vi "OCT.vi"() -> ()   [LabVIEW 2015]
doc: "I. Description:\nThis example demonstrates how to acquire a continuous amount of data (Waveform) using the DAQ device's internal clock.\n\nII. Instructions for Running:\n1. Create an analog input voltage channel.\n2. Set the rate for the sample clock. Additionally, define the sample mode to be continuous.\n3. Call the Start VI to start the acquisition.\n4. Read the waveform data in a loop until the user hits the stop button or an error occurs.\nNote: This example reads data from one or more channels and returns an array of data. Use the Index Array function to access an individual channel of data.\n5. Call the Clear Task VI to clear the Task.\n6. Use the popup dialog box to display an error if any.\n\nIV. I/O Connections Overview:\nMake sure your signal input terminal matches the Physical Channel I/O Control. For further connection information, refer to your hardware reference manual."
uses:
  Type Defs/OCT DAQ Channel Data Type.ctl
  Type Defs/OCT Hardware States.ctl
  Classes/Galvo/Scanning Cluster.ctl
  Classes/DAQ/DAQ Parameters.ctl
  Classes/DAQ/Trigger Source.ctl
  Classes/DAQ/Trigger Slope.ctl
  Classes/DAQ/Clock Control.ctl
  Classes/Galvo/Galvo.lvclass
  Classes/Nufern/Nufern Digital Timing Control.ctl
  Classes/Processing/Intensity/Intensity Processing.lvclass
  Classes/DAQ/DAQ Card Options.ctl
  Classes/Laser/Laser Options.ctl
  Classes/D to A/External Clock Selection.ctl
  Classes/Galvo/Galvo Options.ctl
  Classes/Laser/Axsun/1310/Axsun_1310_SS.lvclass
  Classes/DAQ/ATS9350/ATS9350.lvclass
  Classes/Processing/En Face States.ctl
  Classes/DAQ/DAQ Control Functional Global States.ctl
  Classes/Nufern/Nufern Functional Global States.ctl
  Classes/Processing/Filter/Filter List.ctl
  Classes/Processing/Filter/Kernel Size.ctl
  Classes/Processing/Filter/Std_Dev_Filter/Std. Deviation.lvclass
  Classes/Processing/Filter/Filter.lvclass
  Classes/Processing/Filter/Speckle_Variance_Filter/Speckle Variance Filter.lvclass
  Classes/D to A/No Clock/No Clock.lvclass
  Classes/Galvo/NI Galvo/NI Galvo.lvclass
  Classes/Nufern/Nufern Digital Control Global.vi
  Classes/DAQ/ATS660/ATS660 Class.lvclass
  Classes/DAQ/ATS9462/ATS9462 Class.lvclass
  Classes/Laser/Santec/HSL-2000/HSL-2000.lvclass
  Classes/Laser/Insite/Insight.lvclass
  Classes/D to A/Wavepond/Wavepond.lvclass
  Classes/Galvo/No Galvos/No Galvos.lvclass
  Classes/DAQ/DAQ Class.lvclass
  Classes/Laser/Laser.lvclass
panel:
  out "Enface":T1(plugin-control)
  out "Intensity Graph":sgl[][](graph)
  in  "Nufern Digital Timing Control":T2={"Fire"=FALSE, "Start A-Scan"=0, "Stop A-Scan"=0, "Reps per Fire"=1, "B-Scan Spacing"=1} {"B-Scan Spacing" min=0 max=5000; "Reps per Fire" min=1 max=5000}
  out "Saved Galvo":refnum<class "Galvo.lvclass">
  out "AFG11000 Task":refnum<k21>
  out "Alazar Task":refnum<k21>
  out "Initial DAQ Parameters":T3={"Points Per A-Scan"=1280, "A-Scans Per B-Scan"=832, "Number of B-Scans"=1, "B-Scans Per Transfer"=2, "Trigger Voltage"=140.0, "Trigger Source"=enum."External", "Trigger Slope"=enum."Rising", "Channel"=enum."Channel 1", "Clock"=enum."External Clock", "Bits per Sample"=16.0, "Range"=4.0, "Start Trim"=140, "Stop Trim"=180}
  in  "Laser Status":string
  in  "Scanning Parameters":T8={"Fast Axis Offset"=0.0, "Slow Axis Offset"=0.0, "Slow Axis Amp"=2.0, "Fast Axis Amp"=2.0, "Scan Pattern"=enum."Raster"} {"Fast Axis Amp" max=20 format="%#.2f"; "Slow Axis Amp" max=20 format="%#.2f"; "Slow Axis Offset" max=10 format="%#.2f"; "Fast Axis Offset" max=10 format="%#.2f"}
  out "Log10?":bool
  in  "OCT Hardware States":T9
  out "Background Array":u16[](array[numeric])
  in  "Save Sweep Button":bool
  in  "Data Format":T6
  in  "Save Sweep":bool
  in  "Stop Button":bool
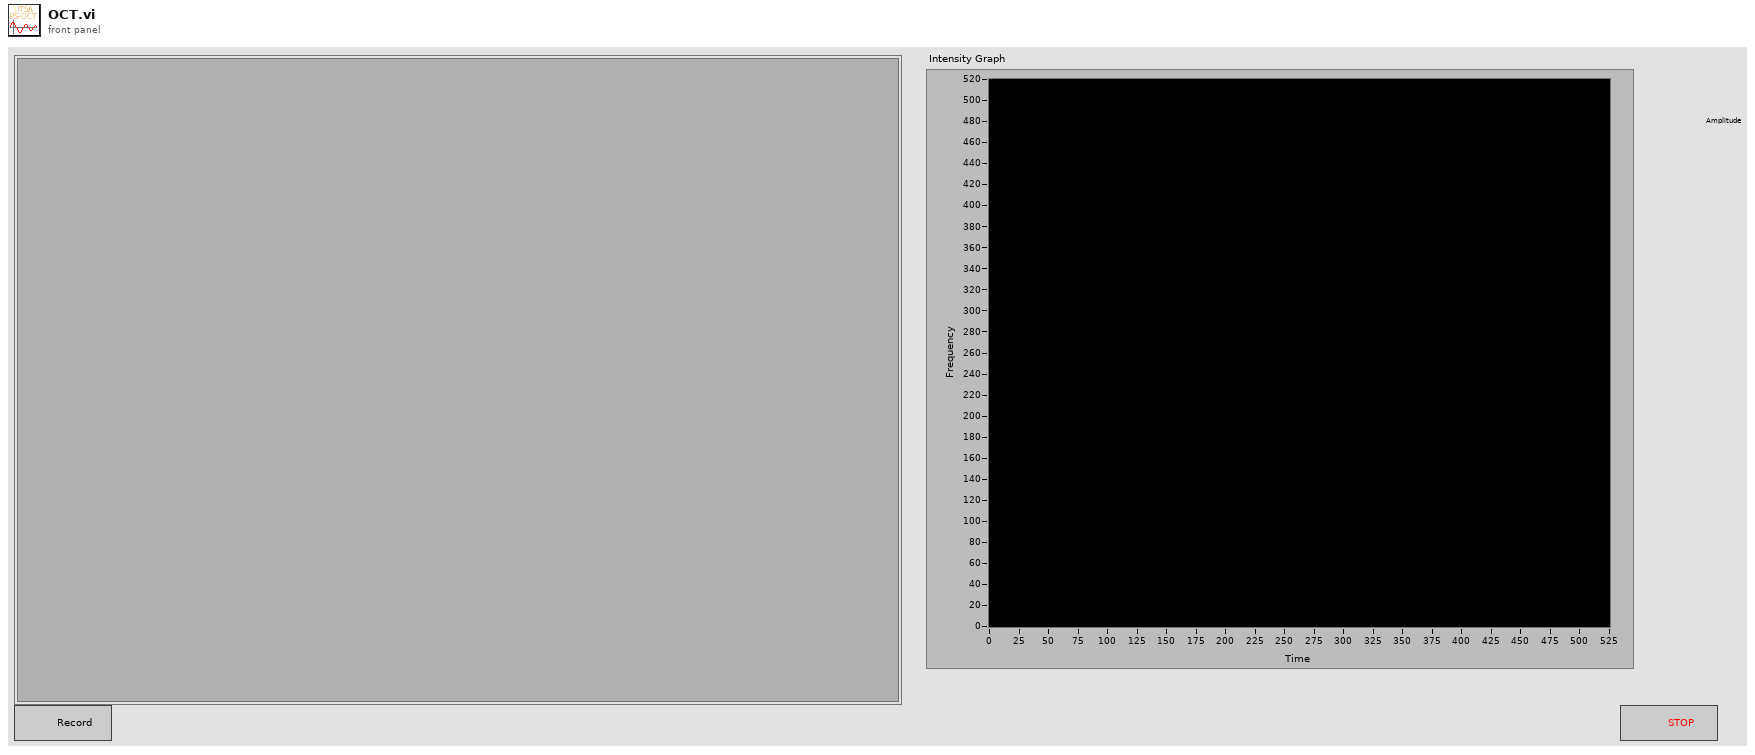
[diagram p1: front panel]
types:
  T1 = typedef "IMAQ Image.ctl" = refnum<image>
  T2 = typedef "Nufern Digital Timing Control.ctl" = cluster{"Fire":bool, "Start A-Scan":u32, "Stop A-Scan":u32, "Reps per Fire":i32, "B-Scan Spacing":i32}
  T3 = typedef "DAQ Class.lvclass/DAQ Parameters.ctl" = cluster{"Points Per A-Scan":u32, "A-Scans Per B-Scan":u32, "Number of B-Scans":u32, "B-Scans Per Transfer":u32, "Trigger Voltage":sgl, "Trigger Source":T4, "Trigger Slope":T5, "Channel":T6, "Clock":T7, "Bits per Sample":dbl, "Range":dbl, "Start Trim":u32, "Stop Trim":u32}
  T4 = typedef "DAQ Class.lvclass/Trigger Source.ctl" = enum16{"External", "Channel A", "Channel B"}
  T5 = typedef "DAQ Class.lvclass/Trigger Slope.ctl" = enum16{"Rising", "Falling"}
  T6 = typedef "OCT DAQ Channel Data Type.ctl" = enum16{"Channel 1", "Channel 2", "Channel 1 and 2"}
  T7 = typedef "DAQ Class.lvclass/Clock Control.ctl" = enum16{"Internal Clock", "External Clock"}
  T8 = typedef "Galvo.lvclass/Scanning Cluster.ctl" = cluster{"Fast Axis Offset":sgl, "Slow Axis Offset":sgl, "Slow Axis Amp":sgl, "Fast Axis Amp":sgl, "Scan Pattern":enum16{"Raster", "Triangle Raster", "Sinusoid Raster"}}
  T9 = typedef "OCT Hardware States.ctl" = enum16{"Acquire Data", "Initialize Laser", "Initialize Galvos", "Startup", "Reset DAQ", "Background Subtraction", "Acquire Background", "Update DAQ Parameters", "Stop", "Set Clock", "Initialize DAQ", "Set Resampling Array", "Save Sweep", "Configure Laser", "128 x 128", "512 x 1", "512 x 512", "Review Data", "Configure Trigger", "Update Galvos", "Update Filter", "Fire Digital Output", "Configure Digital Output", "Save Galvo Settings", "Load Galvo Settings"}
  T10 = typedef "Galvo Options.ctl" = enum16{"NI Galvos", "No Galvos"}
  T11 = typedef "External Clock Selection.ctl" = enum16{"Wavepond", "None"}
  T12 = typedef "Laser Options.ctl" = enum16{"HSL-2000", "Insight_1310", "Axsuin_1310"}
  T13 = typedef "DAQ Class.lvclass/DAQ Card Options.ctl" = enum16{"ATS660", "ATS9462", "ATS9350"}
  T14 = typedef "Nufern Functional Global States.ctl" = enum16{"Init", "Generate Waveform", "Fire", "Shutdown", "Stop"}
  T15 = typedef "DAQ Control Functional Global States.ctl" = enum16{"Status", "Set Processing Finished", "Reset", "Clear", "Set DAQ Finished"}
  T16 = typedef "Kernel Size.ctl" = enum16{"3x3", "5x5", "3x5", "5x3"}
  T17 = typedef "Filter.lvclass/Filter List.ctl" = enum16{"None", "Std. Dev.", "Speckle Variance"}
  T18 = enum32{"Invalid", "Standard", "Closed", "Hidden", "Minimized", "Maximized"}
  T19 = typedef "En Face States.ctl" = enum16{"Reset", "Update", "Get EnFace"}
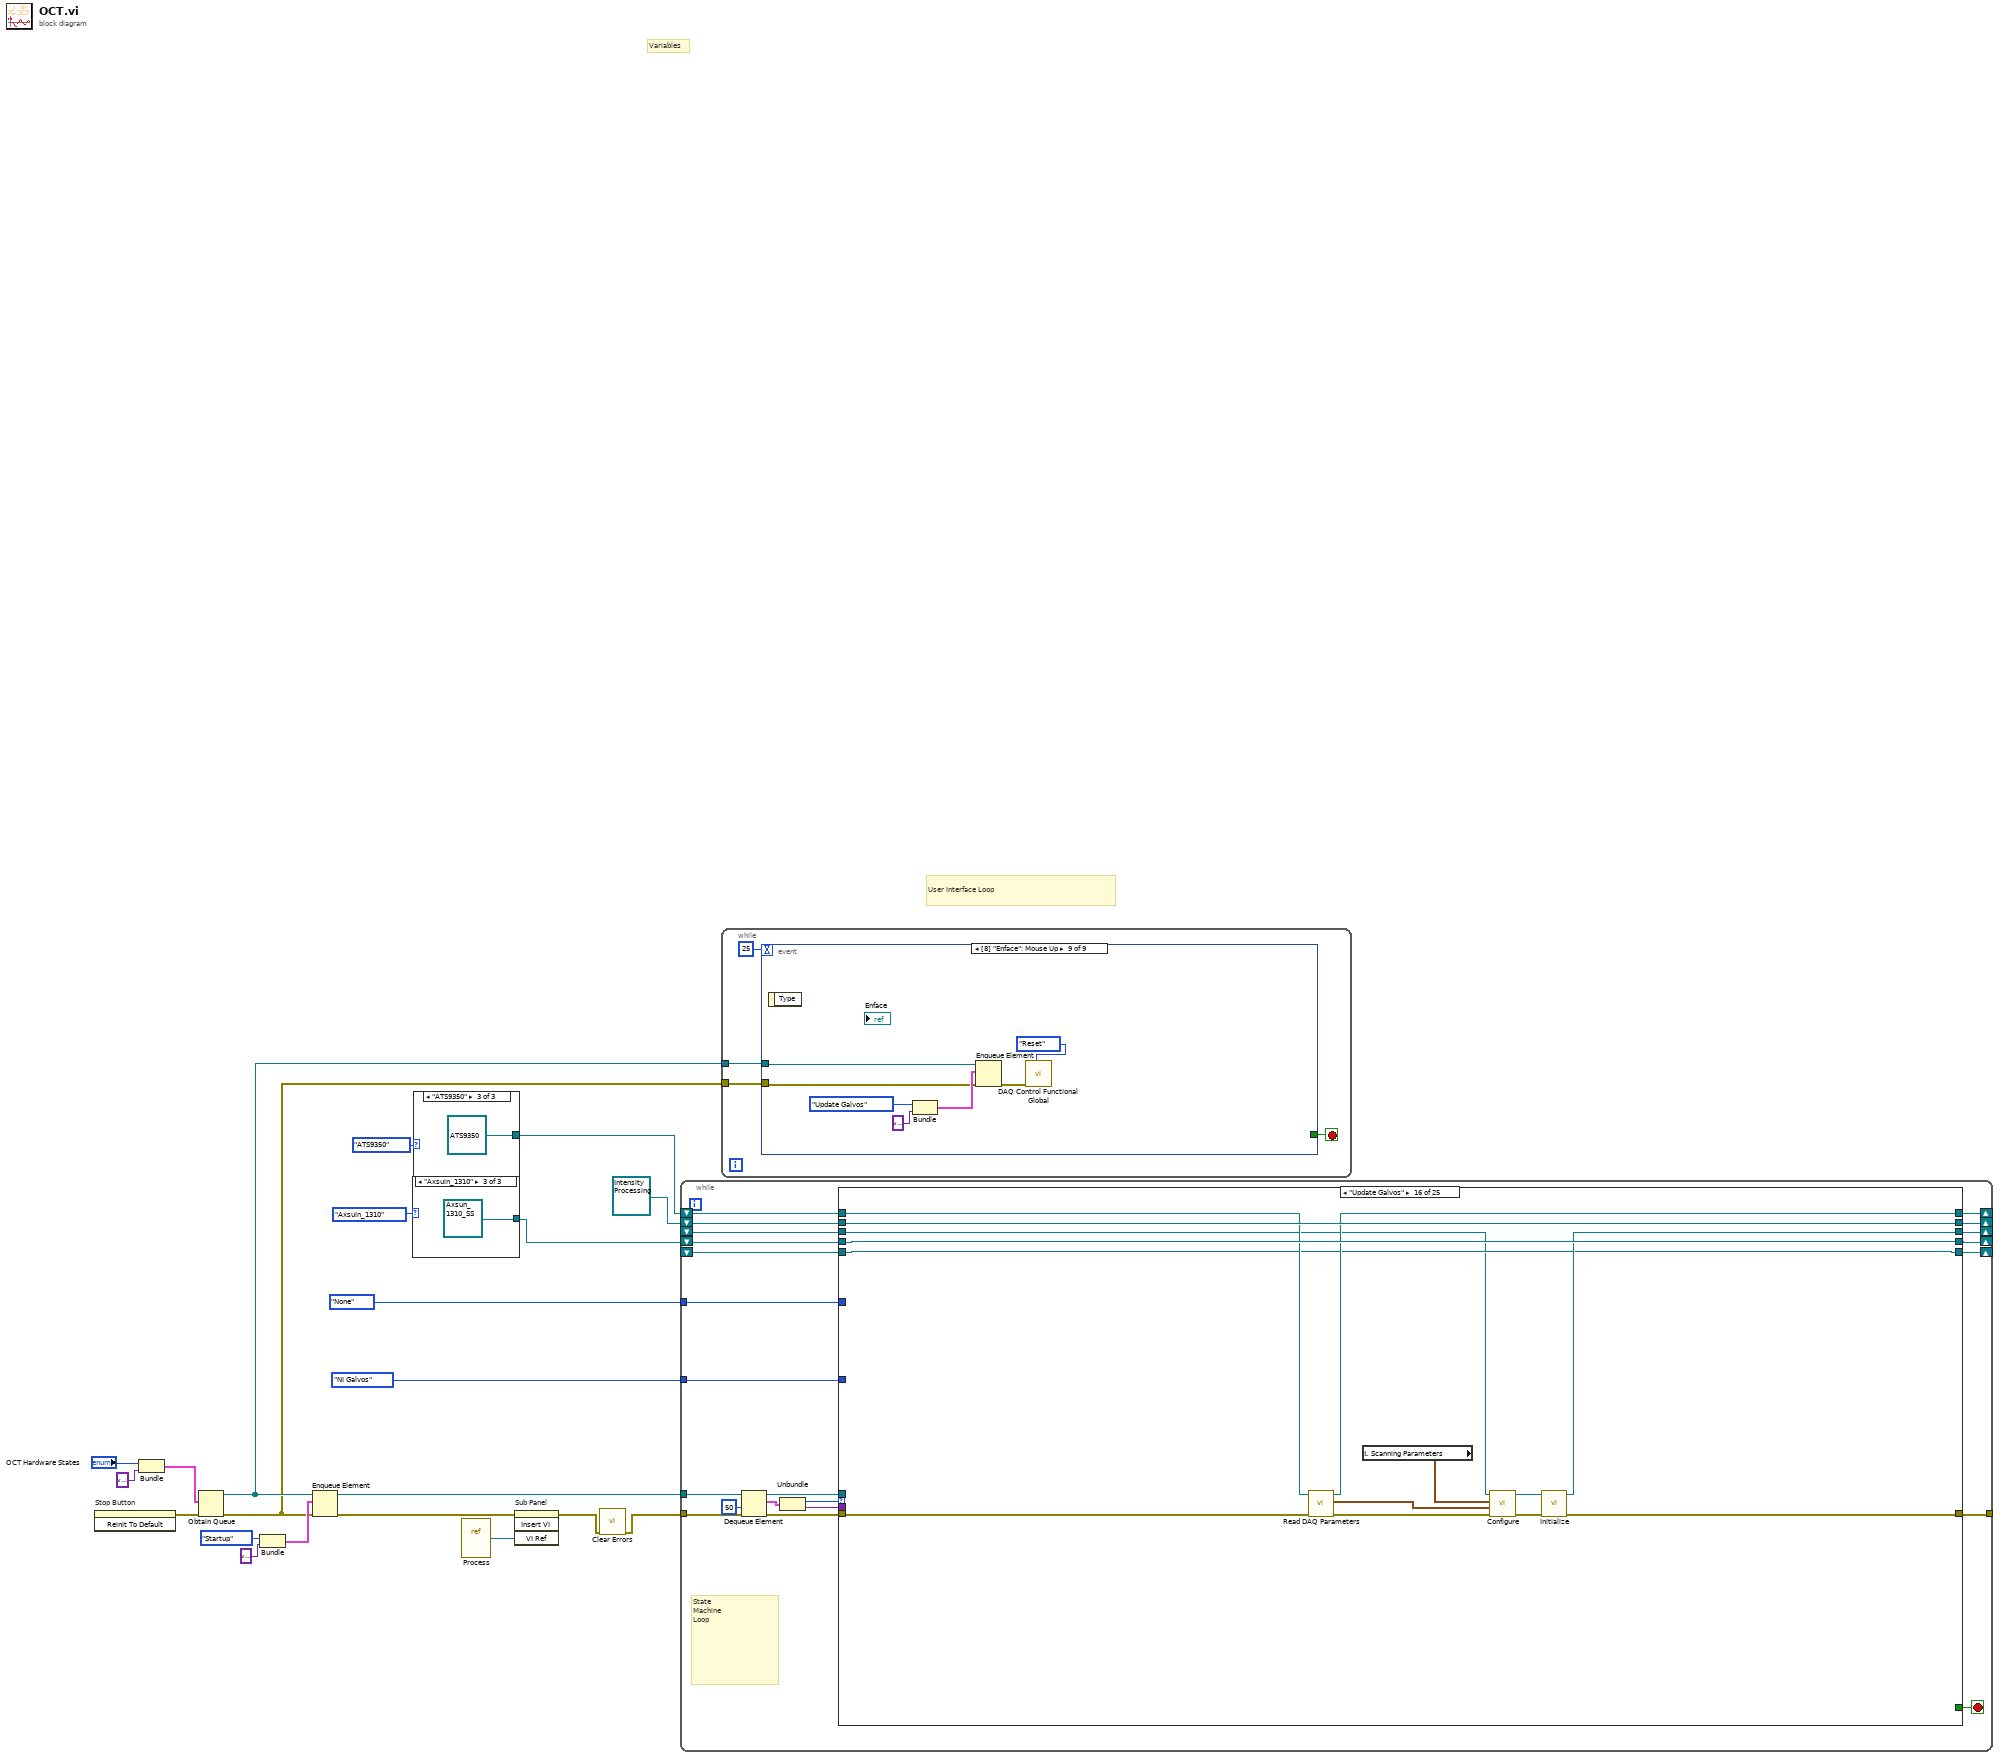
[diagram p0: block diagram]
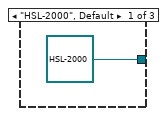
[diagram p2: hidden frame]
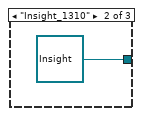
[diagram p3: hidden frame]
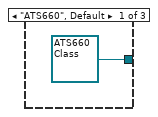
[diagram p4: hidden frame]
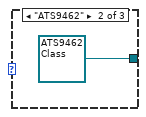
[diagram p5: hidden frame]
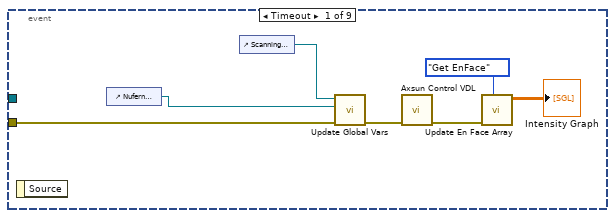
[diagram p6: hidden frame]
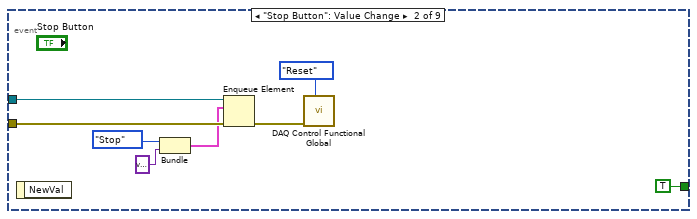
[diagram p7: hidden frame]
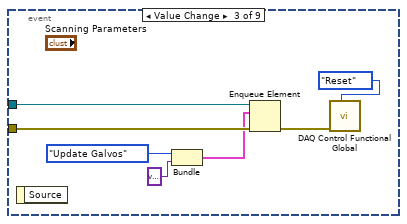
[diagram p8: hidden frame]
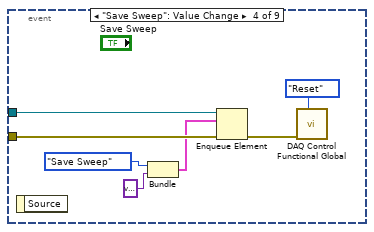
[diagram p9: hidden frame]
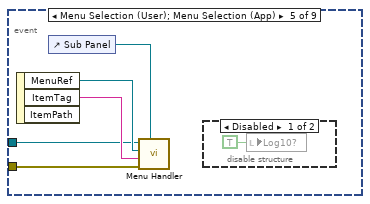
[diagram p10: hidden frame]
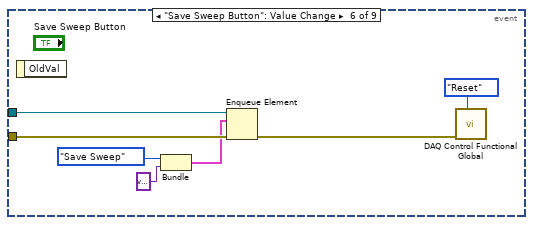
[diagram p12: hidden frame]
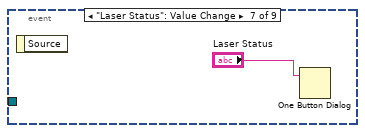
[diagram p13: hidden frame]
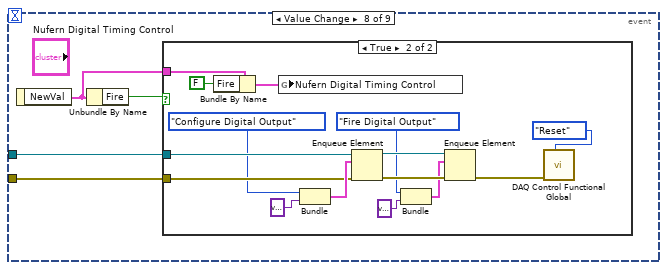
[diagram p14: hidden frame]
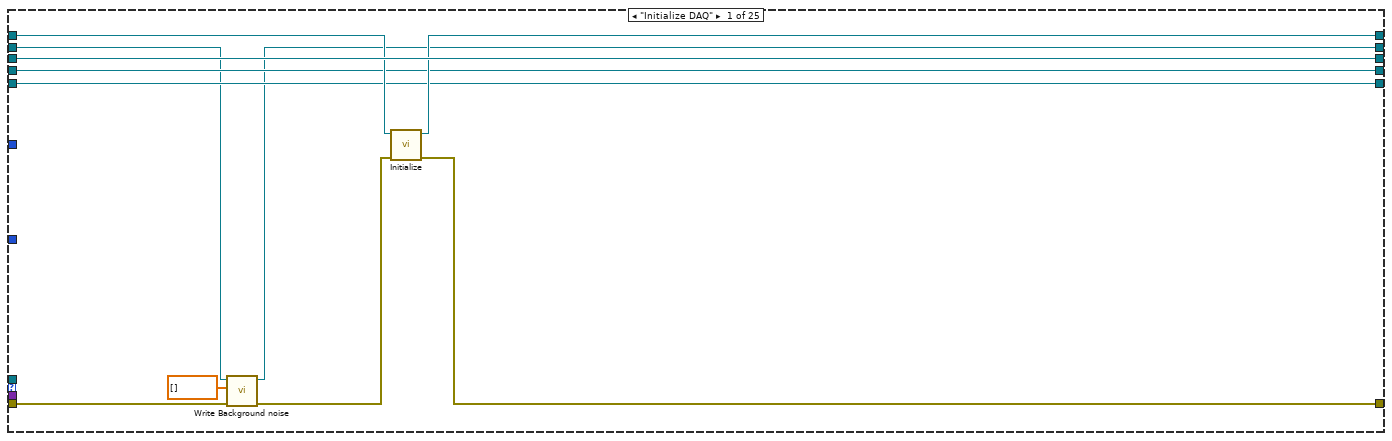
[diagram p16: hidden frame]
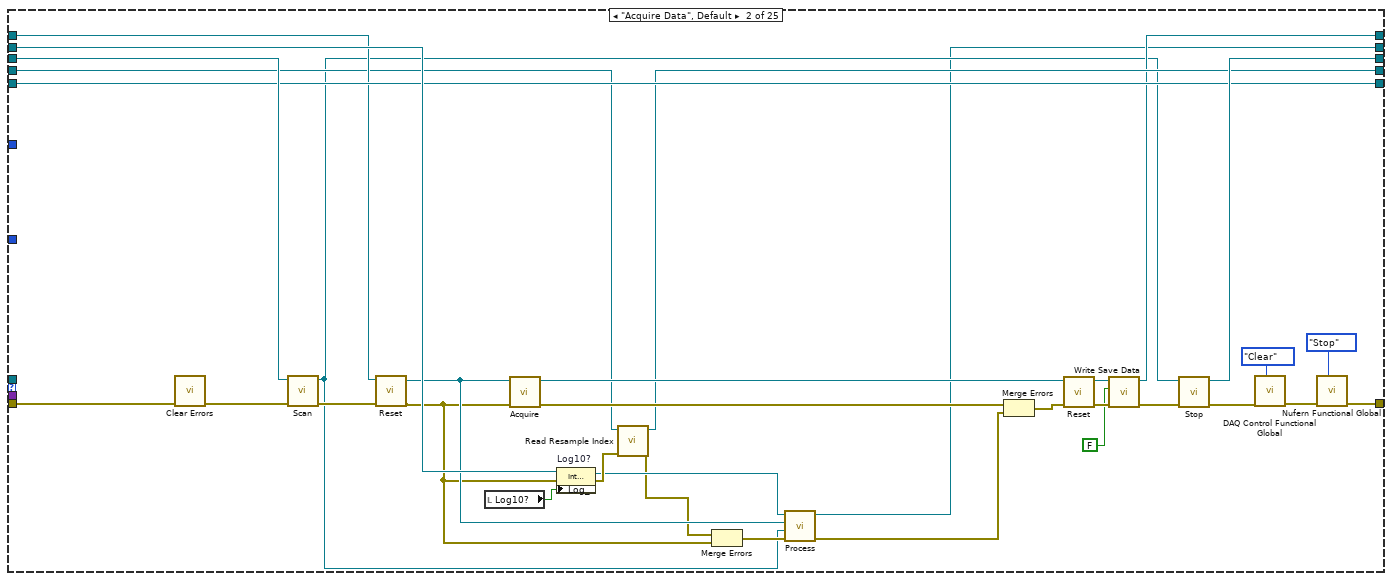
[diagram p17: hidden frame]
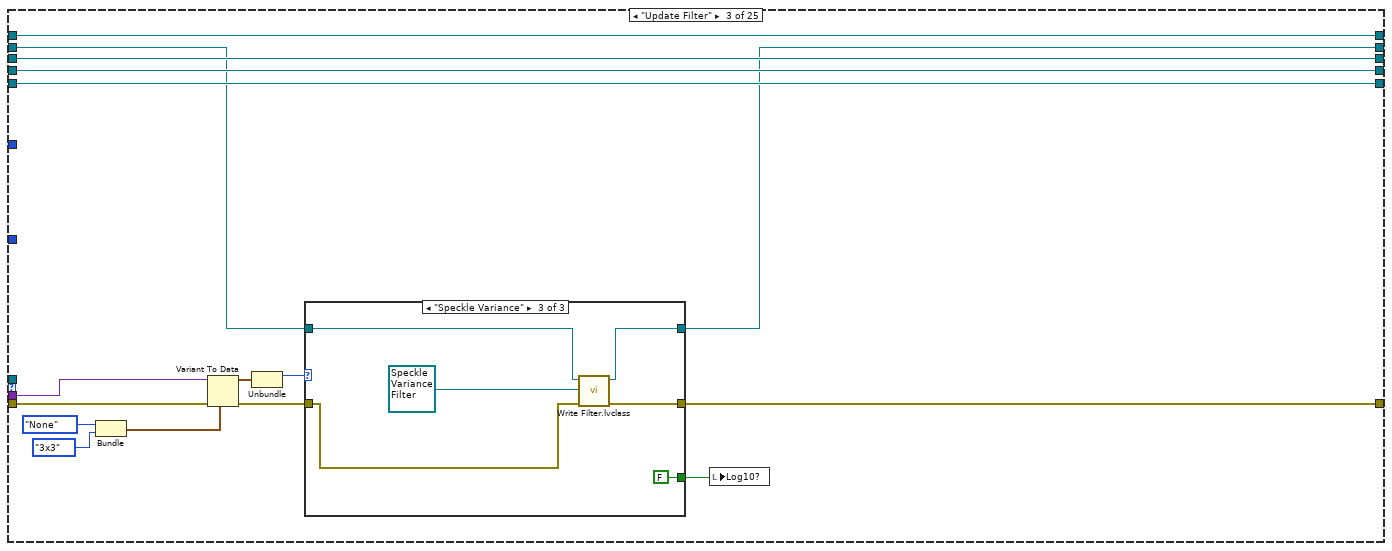
[diagram p18: hidden frame]
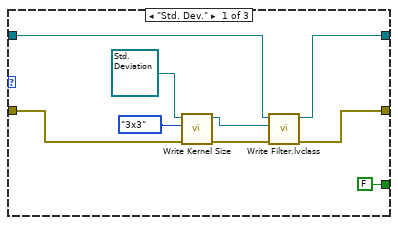
[diagram p19: hidden frame]
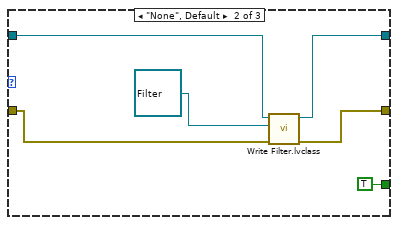
[diagram p20: hidden frame]
diagram:
  # "User Interface Loop"
  # "Variables"
  n1 = invoke on="Stop Button" class="Bool (strict)" method="Reinit To Default"() -> (error out=w14:errorcluster)  [unwired: 3 in, 2 out]
  n2 = Bundle("OCT Hardware States"="OCT Hardware States", variant) -> (w5:cluster{"OCT Hardware States":T9, variant})  [unwired: 1 in]
  n3 = Obtain Queue(element data type=w5, error in (no error)=w14) -> (queue out=w21:refnum<queue>, error out=w1:errorcluster)  [unwired: 3 in, 1 out]
  n4 = Bundle("element"=OCT_Hardware_States."Startup", variant) -> (w3:cluster{"element":T9, variant})  [unwired: 1 in]
  n5 = Enqueue Element(queue=w21, element=w3, error in (no error)=w1) -> (queue out=w18:refnum<queue>, error out=w10:errorcluster)  [unwired: 1 in, 1 out]
  n6 = case shown="\"Axsuin_1310\"" Laser_Options."Axsuin_1310" ("Laser Options") {
    tunnel: [refnum<class "HSL-2000.lvclass"> refnum ("HSL-2000.lvclass") refnum<class "Insight.lvclass"> refnum ("Insight.lvclass") refnum<class "Axsun_1310_SS.lvclass"> refnum ("Axsun_1310_SS.lvclass")] -> w15
    frame "HSL-2000", Default {
    }
    frame "Insight_1310" {
    }
    frame "Axsuin_1310" {
    }
  }
  n7 = case shown="\"ATS9350\"" DAQ_Card_Options."ATS9350" {
    tunnel: [refnum<class "ATS660 Class.lvclass"> refnum ("ATS660 Class.lvclass") refnum<class "ATS9462 Class.lvclass"> refnum ("ATS9462 Class.lvclass") refnum<class "ATS9350.lvclass"> refnum ("ATS9350.lvclass")] -> w19
    frame "ATS660", Default {
    }
    frame "ATS9462" {
    }
    frame "ATS9350" {
    }
  }
  n8 = vi-ref "Process.vi"() -> (w11:refnum<vi>)
  n9 = invoke on="Sub Panel" class="SubPanel" method="Insert VI"(error in=w10, "VI Ref"=w11) -> (error out=w9:errorcluster)  [unwired: 2 in, 3 out]
  n10 = call <vilib>:"Clear Errors.vi"("error in (no error)"=w9) -> ("error out"=w8:errorcluster)  [unwired: 5 in, 1 out]
  n11 = while {
    tunnel: w18 -> [w49]
    tunnel: w8 -> [w44]
    tunnel: [w45] -> _
    shift-right: [w42] -> _
    shift-left: w19 -> [w43]
    shift-right: [w38] -> _
    shift-left: refnum<class "Intensity Processing.lvclass"> refnum ("Intensity Processing.lvclass") -> [w41]
    shift-right: [w37] -> _
    shift-left: _ -> [w40]
    shift-right: [w36] -> _
    shift-left: w15 -> [w39]
    shift-right: [w34] -> _
    shift-left: _ -> [w33]
    tunnel: External_Clock_Selection."None" ("External Clock Options") -> [w32]
    tunnel: Galvo_Options."NI Galvos" ("Galvo Options") -> [w31]
    stop <- w35 stop-if-true
    # "State\nMachine\nLoop"
    n12 = Dequeue Element(queue=w49, timeout in ms (-1)=50, error in (no error)=w44) -> (queue out=w47:refnum<queue>, element=w30:cluster{"OCT Hardware States":T9, variant}, error out=w48:errorcluster)  [unwired: 1 out]
    n13 = Unbundle(w30) -> ("OCT Hardware States"=w29:T9, w28:variant)
    n14 = case shown="\"Update Galvos\"" w29 {
      tunnel: w48 -> [w54 w77 w105 w143 w155 w162 w179 w195 _ w241 w261 _ w336 w367 w369 w401 _ w417 w429 w437 w446 w458 w476 w488 w497]
      tunnel: w47 -> [_ _ _ w144 _ _ _ _ _ _ _ _ w337 w366 _ _ _ _ _ _ _ _ w474 _ _]
      tunnel: [w60 w64 w95 w131 w146 w167 w183 w199 _ w229 w257 _ w307 w365 w376 w408 _ w416 w424 w439 _ w457 w465 w483 w497] -> w45
      tunnel: w43 -> [w58 w81 w109 w139 w148 w163 w180 w196 w208 w232 w258 w306 w341 w364 w372 w404 w413 w421 w432 w445 w455 w463 w482 w484 w502]
      tunnel: [w57 w69 w109 w139 w147 w168 w184 w200 w208 w231 w254 w306 w341 w363 w371 w403 w413 w421 w432 w445 w455 w463 w482 w485 w502] -> w42
      tunnel: w41 -> [w51 w85 w102 w141 w151 w171 w187 w203 w207 w215 w260 w305 w340 w362 w375 w407 w412 w420 w431 w444 w454 w462 w481 w496 w501]
      tunnel: w40 -> [w59 w87 w108 w140 w150 w170 w186 w202 w206 w244 w259 w304 w339 w361 _ w400 w411 w419 w430 w443 w453 w461 w477 w490 _]
      tunnel: w39 -> [w56 w75 w107 w135 w149 w169 w185 w201 w205 w243 w255 w303 w338 w358 w374 w406 w410 w414 w426 w442 w452 w460 w480 w495 w500]
      tunnel: [w52 w62 w101 w141 w151 w171 w187 w203 w207 w214 w260 w305 w340 w362 w375 w407 w412 w420 w431 w444 w454 w462 w481 w496 w501] -> w38
      tunnel: [w59 w86 w108 w140 w150 w170 w186 w202 w206 w244 w259 w304 w339 w361 w373 w405 w411 w419 w430 w443 w453 w461 w477 w490 w498] -> w37
      tunnel: [w56 w74 w107 w135 w149 w169 w185 w201 w205 w243 w255 w303 w338 w357 w374 w406 w410 w415 w425 w442 w452 w460 w480 w495 w500] -> w36
      tunnel: [_ _ _ TRUE _ _ _ _ _ _ _ _ _ _ _ _ _ _ _ _ _ _ _ _ _] -> w35
      tunnel: w33 -> [w55 w84 w106 w137 w145 w166 w182 w198 w204 w242 _ w302 w335 w355 w370 w402 w409 w418 w422 w441 w451 w459 w478 w494 w499]
      tunnel: [w55 w84 w106 w137 w145 w166 w182 w198 w204 w242 w256 w302 w335 w355 w370 w402 w409 w418 w422 w441 w451 w459 w478 w494 w499] -> w34
      tunnel: w32 -> [_ _ _ _ _ _ _ _ _ _ w252 _ _ _ _ _ _ _ _ _ _ _ _ _ _]
      tunnel: w31 -> [_ _ _ _ _ _ _ _ _ _ _ _ _ _ w368 _ _ _ _ _ _ _ _ _ _]
      tunnel: w28 -> [_ _ w104 _ _ _ _ _ _ _ _ _ _ _ _ _ _ _ _ _ _ _ _ _ _]
      frame "Initialize DAQ" {
        n15 = call-dynamic "Write Background noise.vi"("error in (no error)"=w54, "Background noise"=dbl[] [], "Processing in"=w51) -> ("error out"=w53:errorcluster, "Processing out"=w52:refnum<class "Intensity Processing.lvclass">)  [unwired: 7 in]
        n16 = call-dynamic "Initialize.vi"("error in (no error)"=w53, "DAQ Class in"=w58) -> ("error out"=w60:errorcluster, "DAQ Class out"=w57:refnum<class "DAQ Class.lvclass">)  [unwired: 8 in]
      }
      frame "Acquire Data", Default {
        n17 = call <vilib>:"Clear Errors.vi"("error in (no error)"=w77) -> ("error out"=w80:errorcluster)  [unwired: 5 in, 1 out]
        n18 = call-dynamic "Scan.vi"("error in (no error)"=w80, "Galvo in"=w87) -> ("error out"=w83:errorcluster, "Galvo out"=w66:refnum<class "Galvo.lvclass">)  [unwired: 8 in]
        n19 = call-dynamic "Reset.vi"("error in (no error)"=w83, "DAQ Class in"=w81) -> ("error out"=w78:errorcluster, "DAQ Class out"=w82:refnum<class "DAQ Class.lvclass">)  [unwired: 8 in]
        n20 = local read "Log10?"() -> (w89:bool)
        n21 = call-dynamic "Acquire.vi"("error in (no error)"=w78, "DAQ Class in"=w82) -> ("error out"=w92:errorcluster, "DAQ Class out"=w90:refnum<class "DAQ Class.lvclass">)  [unwired: 8 in]
        n22 = property on="Log10?" class="Intensity Processing.lvclass"(reference=w85, error in=w78, "Log_"=w89) -> (reference out=w73:refnum<class "Intensity Processing.lvclass">, error out=w76:errorcluster)
        n23 = call-dynamic "Read Resample Index.vi"("error in (no error)"=w76, "Laser in"=w75) -> ("error out"=w72:errorcluster, "Laser out"=w74:refnum<class "Laser.lvclass">)  [unwired: 7 in, 1 out]
        n24 = Merge Errors(w72, w78) -> (w79:errorcluster)
        n25 = call-dynamic "Process.vi"("error in (no error)"=w79, "Galvo.lvclass"=w66, "DAQ Class.lvclass"=w82, "Intensity Processing in"=w73) -> ("error out"=w61:errorcluster, "Intensity Processing out"=w62:refnum<class "Intensity Processing.lvclass">)  [unwired: 6 in]
        n26 = Merge Errors(w92, w61) -> (w91:errorcluster)
        n27 = call-dynamic "Reset.vi"("error in (no error)"=w91, "DAQ Class in"=w90) -> ("error out"=w71:errorcluster, "DAQ Class out"=w70:refnum<class "DAQ Class.lvclass">)  [unwired: 8 in]
        n28 = call-dynamic "Write Save Data.vi"("error in (no error)"=w71, "Save Data"=FALSE, "DAQ Class in"=w70) -> ("error out"=w68:errorcluster, "DAQ Class out"=w69:refnum<class "DAQ Class.lvclass">)  [unwired: 7 in]
        n29 = call-dynamic "Stop.vi"("error in (no error)"=w68, "Galvo in"=w66) -> ("error out"=w88:errorcluster, "Galvo out"=w86:refnum<class "Galvo.lvclass">)  [unwired: 8 in]
        n30 = call "DAQ Control Functional Global.vi"("State"=DAQ_Control_Functional_Global_States."Clear", "Error In"=w88) -> ("Error Out"=w65:errorcluster)  [unwired: 6 in, 3 out]
        n31 = call "Nufern Functional Global.vi"("Nufern Functional\n Global States"=Nufern_Functional_Global_States."Stop" ("Nufern Functional\n Global States"), "Error In"=w65) -> ("Error Out"=w64:errorcluster)  [unwired: 9 in]
      }
      frame "Update Filter" {
        n32 = Bundle("Filter"=Filter_List."None", "Kernel Size"=Kernel_Size."3x3") -> (w98:cluster{"Filter":T17, "Kernel Size":T16})  [unwired: 1 in]
        n33 = Variant To Data(error in=w105, type=w98, Variant=w104) -> (data=w97:cluster{"Filter":T17, "Kernel Size":T16}, error out=w103:errorcluster)
        n34 = Unbundle(w97) -> ("Filter"=w96:T17)  [unwired: 1 out]
        n35 = case shown="\"Speckle Variance\"" w96 {
          tunnel: w103 -> [w117 w121 w126]
          tunnel: w102 -> [w113 w124 w128]
          tunnel: [w112 w123 w127] -> w101
          tunnel: [w111 w120 w129] -> w95
          tunnel: [FALSE ("Log10?") TRUE ("Log10?") FALSE ("Log10?")] -> w94
          frame "Std. Dev." {
            n36 = call-dynamic "Write Kernel Size.vi"("error in (no error)"=w117, "Kernel Size"=enum16{"3x3", "5x5", "3x5", "5x3"}."3x3", "Std. Deviation in"=refnum<class "Std. Deviation.lvclass"> refnum ("Std. Deviation.lvclass")) -> ("error out"=w115:errorcluster, "Std. Deviation out"=w114:refnum<class "Std. Deviation.lvclass">)  [unwired: 7 in]
            n37 = call-dynamic "Write Filter.lvclass.vi"("error in (no error)"=w115, "Filter.lvclass"=w114, "Processing in"=w113) -> ("error out"=w111:errorcluster, "Processing out"=w112:refnum<class "Intensity Processing.lvclass">)  [unwired: 7 in]
          }
          frame "None", Default {
            n38 = call-dynamic "Write Filter.lvclass.vi"("error in (no error)"=w121, "Filter.lvclass"=refnum<class "Filter.lvclass"> refnum, "Processing in"=w124) -> ("error out"=w120:errorcluster, "Processing out"=w123:refnum<class "Intensity Processing.lvclass">)  [unwired: 7 in]
          }
          frame "Speckle Variance" {
            n39 = call-dynamic "Write Filter.lvclass.vi"("error in (no error)"=w126, "Filter.lvclass"=refnum<class "Speckle Variance Filter.lvclass"> refnum ("Speckle Variance Filter.lvclass"), "Processing in"=w128) -> ("error out"=w129:errorcluster, "Processing out"=w127:refnum<class "Intensity Processing.lvclass">)  [unwired: 7 in]
          }
        }
        n40 = local write "Log10?"(w94) -> ()
      }
      frame "Stop" {
        n41 = Release Queue(queue=w144, error in (no error)=w143) -> (error out=w142:errorcluster)  [unwired: 1 in, 2 out]
        n42 = call-dynamic "Shutdown.vi"("error in (no error)"=w142, "DAQ Class in"=w139) -> ("error out"=w136:errorcluster)  [unwired: 8 in, 1 out]
        n43 = call-dynamic "Shutdown.vi"("error in (no error)"=w136, "Laser in"=w135) -> ("error out"=w132:errorcluster)  [unwired: 8 in, 1 out]
        n44 = local read "AFG11000 Task"() -> (w134:refnum<k21>)
        n45 = local read "Alazar Task"() -> (w133:refnum<k21>)
        n46 = call "Stop Triggers.vi"("Error in"=w132, "Alazar Task"=w133, "AFG11000 Task"=w134) -> ("error out"=w131:errorcluster)  [unwired: 8 in]
      }
      frame "Update DAQ Parameters" {
        n47 = call-dynamic "Update DAQ Parameters.vi"("error in (no error)"=w155, "DAQ Class in"=w148) -> ("error out"=w153:errorcluster, "DAQ Parameters Out"=w152:T3, "DAQ Class out"=w154:refnum<class "DAQ Class.lvclass">)  [unwired: 7 in]
        "Initial DAQ Parameters" <- w152
        n48 = call-dynamic "Write DAQ Parameters.vi"("error in (no error)"=w153, "DAQ Parameters"=w152, "DAQ Class in"=w154) -> ("error out"=w146:errorcluster, "DAQ Class out"=w147:refnum<class "DAQ Class.lvclass">)  [unwired: 7 in]
      }
      frame "128 x 128" {
        w157 = u32 0 ("Stop Trim")
        w158 = u32 200 ("Stop Trim")
        n49 = local read "Initial DAQ Parameters"() -> (w161:T3)
        n50 = Compound Arithmetic op=unknown(u32 256 ("A-Scans Per B-Scan"), w158, w157) -> (w156:u32)
        n51 = Bundle By Name(cluster=w161, "A-Scans Per B-Scan"=w156, "B-Scans Per Transfer"=u32 4, "Number of B-Scans"=u32 256 ("A-Scans Per B-Scan"), "Start Trim"=w158, "Stop Trim"=w157) -> (w165:T3)
        n52 = call-dynamic "Write DAQ Parameters.vi"("error in (no error)"=w162, "DAQ Parameters"=w165, "DAQ Class in"=w163) -> ("error out"=w167:errorcluster, "DAQ Class out"=w168:refnum<class "DAQ Class.lvclass">)  [unwired: 7 in]
      }
      frame "512 x 512" {
        w172 = u32 0 ("Stop Trim")
        w173 = u32 200 ("Stop Trim")
        n53 = Compound Arithmetic op=unknown(u32 512 ("A-Scans Per B-Scan"), w173, w172) -> (w174:u32)
        n54 = local read "Initial DAQ Parameters"() -> (w178:T3)
        n55 = Bundle By Name(cluster=w178, "A-Scans Per B-Scan"=w174, "B-Scans Per Transfer"=u32 4, "Number of B-Scans"=u32 512 ("A-Scans Per B-Scan"), "Start Trim"=w173, "Stop Trim"=w172) -> (w181:T3)
        n56 = call-dynamic "Write DAQ Parameters.vi"("error in (no error)"=w179, "DAQ Parameters"=w181, "DAQ Class in"=w180) -> ("error out"=w183:errorcluster, "DAQ Class out"=w184:refnum<class "DAQ Class.lvclass">)  [unwired: 7 in]
      }
      frame "512 x 1" {
        w189 = u32 200 ("Stop Trim")
        w190 = u32 0 ("Stop Trim")
        n57 = local read "Initial DAQ Parameters"() -> (w192:T3)
        n58 = Compound Arithmetic op=unknown(u32 512 ("A-Scans Per B-Scan"), w190, w189) -> (w188:u32)
        n59 = Bundle By Name(cluster=w192, "A-Scans Per B-Scan"=w188, "B-Scans Per Transfer"=u32 2, "Number of B-Scans"=u32 1, "Stop Trim"=w190, "Start Trim"=w189) -> (w197:T3)
        n60 = call-dynamic "Write DAQ Parameters.vi"("error in (no error)"=w195, "DAQ Parameters"=w197, "DAQ Class in"=w196) -> ("error out"=w199:errorcluster, "DAQ Class out"=w200:refnum<class "DAQ Class.lvclass">)  [unwired: 7 in]
      }
      frame "Background Subtraction" {
      }
      frame "Acquire Background" {
        n61 = call "Display Message to User"("error in (no error)"=w241) -> ("error out"=w240:errorcluster)  [unwired: 9 in, 1 out]
        n62 = local read "Initial DAQ Parameters"() -> (w228:T3)
        n63 = while {
          tunnel: w240 -> [w249]
          tunnel: [w249] -> w217
          stop <- TRUE stop-if-true
          n64 = Wait Until Next ms Multiple(millisecond multiple=u32 250) -> ()  [unwired: 1 out]
        }
        n65 = call-dynamic "Acquire.vi"("error in (no error)"=w240, "DAQ Class in"=w232) -> ("error out"=w239:errorcluster, "DAQ Class out"=w238:refnum<class "DAQ Class.lvclass">)  [unwired: 8 in]
        n66 = Unbundle By Name(w228) -> ("Points Per A-Scan"=w224:u32)
        n67 = call "DAQ Control Functional Global.vi"("State"=DAQ_Control_Functional_Global_States."Reset", "Error In"=w217) -> ("Error Out"=w216:errorcluster)  [unwired: 6 in, 3 out]
        n68 = Merge Errors(w239, w216) -> (w237:errorcluster)
        n69 = call-dynamic "Read Data queue.vi"("error in (no error)"=w237, "DAQ Class in"=w238) -> ("error out"=w235:errorcluster, "Data queue"=w236:refnum<queue>, "DAQ Class out"=w230:refnum<class "DAQ Class.lvclass">)  [unwired: 7 in]
        n70 = Dequeue Element(queue=w236, error in (no error)=w235) -> (element=w226:u16[], error out=w213:errorcluster)  [unwired: 1 in, 2 out]
        n71 = Array Size(array=w226) -> (size(s)=w227:i32)
        n72 = Divide(x=w227, y=w224) -> (x/y=w225:dbl)
        n73 = Reshape Array(w226, w225, w224) -> (w222:u16[][])
        n74 = Initialize Array(0.0 ("element"), w224) -> (w221:dbl[])
        n75 = for {
          N -> [w245]
          tunnel: w222 -> [w246] mode=indexing
          shift-right: [w247] -> w220
          shift-left: w221 -> [w248]
          tunnel: [w245] -> w219
          n76 = Add(x=w246, y=w248) -> (x+y=w247:dbl[])
        }
        n77 = Divide(x=w220, y=w219) -> (x/y=w211:dbl[])
        n78 = Subtract(x=w211, y=32768.0 ("element")) -> (x-y=w210:dbl[])
        n79 = call-dynamic "Write Background noise.vi"("error in (no error)"=w213, "Background noise"=w210, "Processing in"=w215) -> ("error out"=w212:errorcluster, "Processing out"=w214:refnum<class "Intensity Processing.lvclass">)  [unwired: 7 in]
        n80 = call-dynamic "Reset.vi"("error in (no error)"=w212, "DAQ Class in"=w230) -> ("error out"=w233:errorcluster, "DAQ Class out"=w231:refnum<class "DAQ Class.lvclass">)  [unwired: 8 in]
        n81 = call "DAQ Control Functional Global.vi"("State"=DAQ_Control_Functional_Global_States."Clear", "Error In"=w233) -> ("Error Out"=w229:errorcluster)  [unwired: 6 in, 3 out]
      }
      frame "Set Clock" {
        n82 = call "DAQ Control Functional Global.vi"("State"=DAQ_Control_Functional_Global_States."Clear", "Error In"=w261) -> ("Error Out"=w253:errorcluster)  [unwired: 6 in, 3 out]
        n83 = case shown="\"None\"" w252 {
          tunnel: w258 -> [w295 w301]
          tunnel: [w278 w299] -> w257
          tunnel: [w277 refnum<class "No Clock.lvclass"> refnum ("No Clock.lvclass")] -> w256
          tunnel: w255 -> [w263 _]
          tunnel: [w276 w301] -> w254
          tunnel: w253 -> [w266 w299]
          frame "Wavepond", Default {
            n84 = call-dynamic "Write Path to resampled Clock.vi"("error in (no error)"=w266, "Path to resampled Clock"=path "c:/software/wavepond.txt", "Wavepond in"=refnum<class "Wavepond.lvclass"> refnum ("Wavepond.lvclass")) -> ("error out"=w269:errorcluster, "Wavepond out"=w270:refnum<class "Wavepond.lvclass">)  [unwired: 7 in]
            n85 = call-dynamic "Write Path to AFG_.exe.vi"("error in (no error)"=w269, "Path to AFG*.exe"=path "c:/software" ("Path to resampled Clock"), "Wavepond in"=w270) -> ("error out"=w267:errorcluster, "Wavepond out"=w265:refnum<class "Wavepond.lvclass">)  [unwired: 7 in]
            n86 = call "Compute 1 A-Scan Parameters.vi"("error in (no error)"=w267, "Laser In"=w263, "DAQ Class.lvclass"=w295) -> ("error out"=w296:errorcluster, "DAQ Parameters"=w294:T3, "DAQ Class.lvclass 2"=w280:refnum<class "DAQ Class.lvclass">)  [unwired: 6 in]
            n87 = Bundle By Name(cluster=w294, "Trigger Source"=Trigger_Source."External", "Trigger Slope"=Trigger_Slope."Rising", "Trigger Voltage"=sgl 180.0, "Channel"=OCT_DAQ_Channel_Data_Type."Channel 2", "Clock"=Clock_Control."Internal Clock") -> (w288:T3)
            n88 = call-dynamic "Write DAQ Parameters.vi"("error in (no error)"=w296, "DAQ Parameters"=w288, "DAQ Class in"=w280) -> ("error out"=w283:errorcluster, "DAQ Class out"=w282:refnum<class "DAQ Class.lvclass">)  [unwired: 7 in]
            n89 = Unbundle By Name(w288) -> ("Points Per A-Scan"=w286:u32)
            n90 = call-dynamic "Reset.vi"("error in (no error)"=w283, "DAQ Class in"=w282) -> ("error out"=w285:errorcluster, "DAQ Class out"=w284:refnum<class "DAQ Class.lvclass">)  [unwired: 8 in]
            n91 = call-dynamic "Acquire.vi"("error in (no error)"=w285, "DAQ Class in"=w284) -> ("error out"=w297:errorcluster, "DAQ Class out"=w298:refnum<class "DAQ Class.lvclass">)  [unwired: 8 in]
            n92 = call-dynamic "Get Last Buffer.vi"("error in (no error)"=w297, "DAQ Class in"=w298) -> ("error out"=w292:errorcluster, "Last Buffer"=w287:u16[], "DAQ Class out"=w291:refnum<class "DAQ Class.lvclass">)  [unwired: 7 in]
            n93 = Array Subset(array=w287, length=w286) -> (w281:u16[])  [unwired: 1 in]
            n94 = call-dynamic "Reset.vi"("error in (no error)"=w292, "DAQ Class in"=w291) -> ("error out"=w275:errorcluster, "DAQ Class out"=w276:refnum<class "DAQ Class.lvclass">)  [unwired: 8 in]
            n95 = call-dynamic "Compute Clock.vi"("k-space signal in"=w281, "error in (no error)"=w275, "Laser.lvclass"=w263, "DAQ Class.lvclass"=w276, "Wavepond in"=w265) -> ("error out"=w272:errorcluster, "Wavepond out"=w279:refnum<class "Wavepond.lvclass">)  [unwired: 5 in]
            n96 = call-dynamic "Run.vi"("error in (no error)"=w272, "Wavepond in"=w279) -> ("error out"=w278:errorcluster, "Wavepond out"=w277:refnum<class "Wavepond.lvclass">)  [unwired: 8 in]
          }
          frame "None" {
          }
        }
      }
      frame "Set Resampling Array" {
      }
      frame "Startup" {
        n97 = Bundle("element"=OCT_Hardware_States."Initialize Laser", variant) -> (w322:cluster{"element":T9, variant})  [unwired: 1 in]
        n98 = Enqueue Element(queue=w337, element=w322, error in (no error)=w336) -> (queue out=w333:refnum<queue>, error out=w334:errorcluster)  [unwired: 1 in, 1 out]
        n99 = Bundle("element"=OCT_Hardware_States."Configure Trigger", variant) -> (w321:cluster{"element":T9, variant})  [unwired: 1 in]
        n100 = Enqueue Element(queue=w333, element=w321, error in (no error)=w334) -> (queue out=w331:refnum<queue>, error out=w332:errorcluster)  [unwired: 1 in, 1 out]
        n101 = local write "Stop Button"(FALSE ("Sweep Ready for saving")) -> ()
        n102 = Bundle("element"=OCT_Hardware_States."Initialize DAQ", variant) -> (w318:cluster{"element":T9, variant})  [unwired: 1 in]
        n103 = Enqueue Element(queue=w331, element=w318, error in (no error)=w332) -> (queue out=w345:refnum<queue>, error out=w344:errorcluster)  [unwired: 1 in, 1 out]
        n104 = Bundle("element"=OCT_Hardware_States."Set Clock", variant) -> (w316:cluster{"element":T9, variant})  [unwired: 1 in]
        n105 = Enqueue Element(queue=w345, element=w316, error in (no error)=w344) -> (queue out=w343:refnum<queue>, error out=w342:errorcluster)  [unwired: 1 in, 1 out]
        n106 = Bundle("element"=OCT_Hardware_States."Update DAQ Parameters", variant) -> (w314:cluster{"element":T9, variant})  [unwired: 1 in]
        n107 = Enqueue Element(queue=w343, element=w314, error in (no error)=w342) -> (queue out=w351:refnum<queue>, error out=w350:errorcluster)  [unwired: 1 in, 1 out]
        n108 = Bundle("element"=OCT_Hardware_States."Initialize Galvos", variant) -> (w312:cluster{"element":T9, variant})  [unwired: 1 in]
        n109 = Enqueue Element(queue=w351, element=w312, error in (no error)=w350) -> (queue out=w347:refnum<queue>, error out=w346:errorcluster)  [unwired: 1 in, 1 out]
        n110 = Bundle("element"=OCT_Hardware_States."Acquire Data", variant) -> (w310:cluster{"element":T9, variant})  [unwired: 1 in]
        n111 = Enqueue Element(queue=w347, element=w310, error in (no error)=w346) -> (error out=w308:errorcluster)  [unwired: 1 in, 2 out]
        n112 = call "Nufern Functional Global.vi"("Nufern Functional\n Global States"=Nufern_Functional_Global_States."Init" ("Nufern Functional\n Global States"), "Error In"=w308) -> ("Error Out"=w307:errorcluster)  [unwired: 9 in]
        "Log10?" <- TRUE ("Log10?")
      }
      frame "Save Sweep" {
        n113 = Bundle("element"=OCT_Hardware_States."Acquire Data", variant) -> (w352:cluster{"element":T9, variant})  [unwired: 1 in]
        n114 = Enqueue Element(queue=w366, element=w352, error in (no error)=w367) -> (error out=w360:errorcluster)  [unwired: 1 in, 2 out]
        n115 = call-dynamic "Read Resample Index.vi"("error in (no error)"=w360, "Laser in"=w358) -> ("error out"=w359:errorcluster, "Resample Index"=w356:u32[], "Laser out"=w357:refnum<class "Laser.lvclass">)  [unwired: 7 in]
        n116 = call-dynamic "Save.vi"("error in (no error)"=w359, "Resampling Array"=w356, "DAQ Class in"=w364) -> ("error out"=w365:errorcluster, "DAQ Class out"=w363:refnum<class "DAQ Class.lvclass">)  [unwired: 7 in]
      }
      frame "Initialize Galvos" {
        n117 = case shown="\"NI Galvos\", Default" w368 {
          tunnel: [w388 w393] -> w376
          tunnel: [w385 refnum<class "No Galvos.lvclass"> refnum ("No Galvos.lvclass")] -> w373
          tunnel: w372 -> [w384 w394]
          tunnel: [w383 w394] -> w371
          tunnel: w369 -> [w381 w393]
          frame "NI Galvos", Default {
            n118 = call-dynamic "Set Channels.vi"("error in (no error)"=w381, "Trigger Source"=tag "/Dev1/PFI7", "Analog Output"=tag "Dev1/ao0:1", "NI Galvo in"=refnum<class "NI Galvo.lvclass"> refnum ("NI Galvo.lvclass")) -> ("error out"=w380:errorcluster, "NI Galvo out"=w378:refnum<class "NI Galvo.lvclass">)  [unwired: 6 in]
            n119 = call-dynamic "Read DAQ Parameters.vi"("error in (no error)"=w380, "DAQ Class in"=w384) -> ("error out"=w386:errorcluster, "DAQ Parameters"=w387:T3, "DAQ Class out"=w383:refnum<class "DAQ Class.lvclass">)  [unwired: 7 in]
            n120 = local read "Scanning Parameters"() -> (w391:T8)
            n121 = call-dynamic "Configure.vi"("error in (no error)"=w386, "DAQ Parameters"=w387, "Scanning Parameters"=w391, "NI Galvo in"=w378) -> ("error out"=w390:errorcluster, "NI Galvo out"=w389:refnum<class "NI Galvo.lvclass">)  [unwired: 6 in]
            n122 = call-dynamic "Initialize.vi"("error in (no error)"=w390, "NI Galvo in"=w389) -> ("error out"=w388:errorcluster, "NI Galvo out"=w385:refnum<class "NI Galvo.lvclass">)  [unwired: 8 in]
          }
          frame "No Galvos" {
          }
        }
      }
      frame "Update Galvos" {
        n123 = call-dynamic "Read DAQ Parameters.vi"("error in (no error)"=w401, "DAQ Class in"=w404) -> ("error out"=w395:errorcluster, "DAQ Parameters"=w396:T3, "DAQ Class out"=w403:refnum<class "DAQ Class.lvclass">)  [unwired: 7 in]
        n124 = local read "Scanning Parameters"() -> (w399:T8)
        n125 = call-dynamic "Configure.vi"("error in (no error)"=w395, "DAQ Parameters"=w396, "Scanning"=w399, "Galvo in"=w400) -> ("error out"=w398:errorcluster, "Galvo out"=w397:refnum<class "Galvo.lvclass">)  [unwired: 6 in]
        n126 = call-dynamic "Initialize.vi"("error in (no error)"=w398, "Galvo in"=w397) -> ("error out"=w408:errorcluster, "Galvo out"=w405:refnum<class "Galvo.lvclass">)  [unwired: 8 in]
      }
      frame "Reset DAQ" {
      }
      frame "Configure Laser" {
        n127 = call-dynamic "Configure.vi"("error in (no error)"=w417, "Laser in"=w414) -> ("error out"=w416:errorcluster, "Laser out"=w415:refnum<class "Laser.lvclass">)  [unwired: 8 in]
      }
      frame "Initialize Laser" {
        n128 = call-dynamic "Init.vi"("error in (no error)"=w429, "Laser in"=w426) -> ("error out"=w427:errorcluster, "Laser out"=w428:refnum<class "Laser.lvclass">)  [unwired: 8 in]
        n129 = call-dynamic "Read Status.vi"("error in (no error)"=w427, "Laser in"=w428) -> ("error out"=w424:errorcluster, "Status"=w423:string, "Laser out"=w425:refnum<class "Laser.lvclass">)  [unwired: 7 in]
        n130 = local write "Laser Status"(w423) -> ()
      }
      frame "Review Data" {
        w440 = TRUE ("Auto Dispose Reference")
        n131 = vi-ref "Post-Processing VI Bin Files.vi"() -> (w438:refnum<vi>)
        n132 = invoke class="VI" method="FP.Open"(reference=w438, error in=w437, "Activate"=TRUE ("Activate?"), "State"=T18."Standard") -> (reference out=w435:refnum<vi>, error out=w436:errorcluster)  [unwired: 1 in, 3 out]
        n133 = invoke class="VI" method="Run VI"(reference=w435, error in=w436, "Wait until done"=w440, "Auto Dispose Ref"=w440) -> (error out=w439:errorcluster)  [unwired: 1 in, 4 out]
      }
      frame "Configure Trigger" {
        n134 = call "Trigger Maker from TTL Input.vi"("Trigger Delay Alazar"=u32 145, "Error in"=w446, "Master Trigger In from Laser (TTL)"=tag "/Dev1/PFI8") -> ("Alazar Task"=→"Alazar Task":refnum<k21>, "AFG11000 Task"=→"AFG11000 Task":refnum<k21>)  [unwired: 6 in, 1 out]
      }
      frame "Fire Digital Output" {
        n135 = call "Nufern Functional Global.vi"("Nufern Functional\n Global States"=Nufern_Functional_Global_States."Fire" ("Nufern Functional\n Global States"), "Error In"=w458) -> ("Error Out"=w457:errorcluster)  [unwired: 9 in]
      }
      frame "Configure Digital Output" {
        n136 = Bundle("element"=OCT_Hardware_States."Save Galvo Settings", variant) -> (w471:cluster{"element":T9, variant})  [unwired: 1 in]
        n137 = Enqueue Element(queue=w474, element=w471, error in (no error)=w476) -> (queue out=w469:refnum<queue>, error out=w475:errorcluster)  [unwired: 1 in, 1 out]
        n138 = local read "Nufern Digital Timing Control"() -> (w464:T2)
        n139 = call "Nufern Functional Global.vi"("Galvo.lvclass"=w477, "Nufern Functional\n Global States"=Nufern_Functional_Global_States."Generate Waveform" ("Nufern Functional\n Global States"), "Error In"=w475, "Nufern Digital Timing Control"=w464) -> ("Error Out"=w470:errorcluster)  [unwired: 7 in]
        n140 = Bundle("element"=OCT_Hardware_States."Update Galvos", variant) -> (w466:cluster{"element":T9, variant})  [unwired: 1 in]
        n141 = Enqueue Element(queue=w469, element=w466, error in (no error)=w470) -> (error out=w465:errorcluster)  [unwired: 1 in, 2 out]
      }
      frame "Save Galvo Settings" {
        n142 = call-dynamic "Read DAQ Parameters.vi"("error in (no error)"=w488, "DAQ Class in"=w484) -> ("error out"=w487:errorcluster, "DAQ Parameters"=w486:T3, "DAQ Class out"=w485:refnum<class "DAQ Class.lvclass">)  [unwired: 7 in]
        n143 = local read "Scanning Parameters"() -> (w493:T8)
        n144 = call-dynamic "Configure.vi"("error in (no error)"=w487, "DAQ Parameters"=w486, "Scanning"=w493, "Galvo in"=w490) -> ("error out"=w492:errorcluster, "Galvo out"=w491:refnum<class "Galvo.lvclass">)  [unwired: 6 in]
        n145 = call-dynamic "Initialize.vi"("error in (no error)"=w492, "Galvo in"=w491) -> ("error out"=w483:errorcluster, "Galvo out"=→"Saved Galvo":refnum<class "Galvo.lvclass">)  [unwired: 8 in]
      }
      frame "Load Galvo Settings" {
        n146 = local read "Saved Galvo"() -> (w498:refnum<class "Galvo.lvclass">)
      }
    }
  }
  n147 = while {
    tunnel: w21 -> [w506]
    tunnel: w1 -> [w505]
    stop <- w503 stop-if-true
    n148 = event shown="[8] \"Enface\": Mouse Up" {
      selector: _ -> [_ _ _ _ _ _ _ _ _]
      dyn-events: _ -> [_ _ _ _ _ _ _ _ _]
      timeout: 25 -> [_ _ _ _ _ _ _ _ _]
      tunnel: w506 -> [_ w520 w526 w533 w536 w545 _ w552 w572]
      tunnel: w505 -> [w513 w521 w527 w534 w540 w547 _ w553 w571]
      tunnel: [_ TRUE _ _ _ _ _ _ _] -> w503
      event Timeout {
        n149 = event-data() -> ()  [unwired: 1 in, 1 out]
        n150 = control-ref of="Nufern Digital Timing Control"() -> (w510:refnum<vi>)
        n151 = control-ref of="Scanning Parameters"() -> (w511:refnum<vi>)
        n152 = call "Update Global Vars.vi"("Error In"=w513, "Nufern Digital Timing Control 2"=w510, "Scanning Parameters"=w511) -> ("Error Out"=w512:errorcluster)  [unwired: 8 in]
        n153 = call "Axsun Control VDL.vi"("error in (no error)"=w512) -> ("error in (no error) 2"=w509:errorcluster)  [unwired: 10 in]
        n154 = call "Update En Face Array.vi"("State"=En_Face_States."Get EnFace", "Error In"=w509) -> ("Array out"=→"Intensity Graph":sgl[][])  [unwired: 7 in, 2 out]
      }
      event "Stop Button": Value Change {
        n155 = event-data() -> ()  [unwired: 1 in, 1 out]
        n156 = Bundle("element"=OCT_Hardware_States."Stop", variant) -> (w514:cluster{"element":T9, variant})  [unwired: 1 in]
        n157 = Enqueue Element(queue=w520, element=w514, error in (no error)=w521) -> (error out=w519:errorcluster)  [unwired: 1 in, 2 out]
        n158 = call "DAQ Control Functional Global.vi"("State"=DAQ_Control_Functional_Global_States."Reset", "Error In"=w519) -> ()  [unwired: 6 in, 4 out]
      }
      event Value Change {
        n159 = event-data() -> ()  [unwired: 1 in, 1 out]
        n160 = Bundle("element"=OCT_Hardware_States."Update Galvos", variant) -> (w522:cluster{"element":T9, variant})  [unwired: 1 in]
        n161 = Enqueue Element(queue=w526, element=w522, error in (no error)=w527) -> (error out=w528:errorcluster)  [unwired: 1 in, 2 out]
        n162 = call "DAQ Control Functional Global.vi"("State"=DAQ_Control_Functional_Global_States."Reset", "Error In"=w528) -> ()  [unwired: 6 in, 4 out]
      }
      event "Save Sweep": Value Change {
        n163 = event-data() -> ()  [unwired: 1 in, 1 out]
        n164 = Bundle("element"=OCT_Hardware_States."Save Sweep", variant) -> (w529:cluster{"element":T9, variant})  [unwired: 1 in]
        n165 = Enqueue Element(queue=w533, element=w529, error in (no error)=w534) -> (error out=w532:errorcluster)  [unwired: 1 in, 2 out]
        n166 = call "DAQ Control Functional Global.vi"("State"=DAQ_Control_Functional_Global_States."Reset", "Error In"=w532) -> ()  [unwired: 6 in, 4 out]
      }
      event Menu Selection (User); Menu Selection (App) {
        n167 = event-data() -> ("MenuRef"=w539:refnum<k9>, "ItemTag"=w538:string)  [unwired: 1 in, 1 out]
        n168 = control-ref of="Sub Panel"() -> (w537:refnum<vi>)
        n169 = call "Menu Handler.vi"("Sub Panel"=w537, "error in (no error)"=w540, "ItemTag"=w538, "Menu in"=w539, "queue out"=w536) -> ()  [unwired: 5 in, 2 out]
        n170 = disable-structure shown="Disabled" {
          frame Disabled {
            n171 = local write "Log10?"(TRUE ("Log10?")) -> ()
          }
          frame Enabled {
          }
        }
      }
      event "Save Sweep Button": Value Change {
        n172 = event-data() -> ()  [unwired: 1 in, 1 out]
        n173 = Bundle("element"=OCT_Hardware_States."Save Sweep", variant) -> (w542:cluster{"element":T9, variant})  [unwired: 1 in]
        n174 = Enqueue Element(queue=w545, element=w542, error in (no error)=w547) -> (error out=w546:errorcluster)  [unwired: 1 in, 2 out]
        n175 = call "DAQ Control Functional Global.vi"("State"=DAQ_Control_Functional_Global_States."Reset", "Error In"=w546) -> ()  [unwired: 6 in, 4 out]
      }
      event "Laser Status": Value Change {
        n176 = event-data() -> ()  [unwired: 1 in, 1 out]
        n177 = One Button Dialog(message="Laser Status") -> ()  [unwired: 1 in, 1 out]
      }
      event Value Change {
        n178 = event-data() -> ("NewVal"=w550:T2)  [unwired: 1 in]
        n179 = Unbundle By Name(w550) -> ("Fire"=w551:bool)
        n180 = case shown="True" w551 {
          tunnel: w553 -> [_ w566]
          tunnel: w552 -> [_ w568]
          tunnel: w550 -> [_ w556]
          frame False {
          }
          frame True {
            n181 = Bundle By Name(cluster=w556, "Fire"=FALSE) -> (w555:T2)
            n182 = global write "Nufern Digital Control Global.vi" "Nufern Digital Timing Control"(w555) -> ()
            n183 = Bundle("element"=OCT_Hardware_States."Configure Digital Output", variant) -> (w567:cluster{"element":T9, variant})  [unwired: 1 in]
            n184 = Enqueue Element(queue=w568, element=w567, error in (no error)=w566) -> (queue out=w563:refnum<queue>, error out=w562:errorcluster)  [unwired: 1 in, 1 out]
            n185 = Bundle("element"=OCT_Hardware_States."Fire Digital Output", variant) -> (w561:cluster{"element":T9, variant})  [unwired: 1 in]
            n186 = Enqueue Element(queue=w563, element=w561, error in (no error)=w562) -> (error out=w558:errorcluster)  [unwired: 1 in, 2 out]
            n187 = call "DAQ Control Functional Global.vi"("State"=DAQ_Control_Functional_Global_States."Reset", "Error In"=w558) -> ()  [unwired: 6 in, 4 out]
          }
        }
      }
      event "Enface": Mouse Up {
        n188 = event-data() -> ()  [unwired: 1 in, 1 out]
        n189 = Bundle("element"=OCT_Hardware_States."Update Galvos", variant) -> (w573:cluster{"element":T9, variant})  [unwired: 1 in]
        n190 = Enqueue Element(queue=w572, element=w573, error in (no error)=w571) -> (error out=w570:errorcluster)  [unwired: 1 in, 2 out]
        n191 = call "DAQ Control Functional Global.vi"("State"=DAQ_Control_Functional_Global_States."Reset", "Error In"=w570) -> ()  [unwired: 6 in, 4 out]
      }
    }
  }
